vi "New Folder.vi"(8 "error in (no error)":errorcluster, 11 "folder name":string) -> (0 "error out":errorcluster, 3 "Folder Item out":refnum<class "Folder Item.lvclass">)   [LabVIEW 2020, in "BetterDragAndDropDemo.lvlib" / "Folder Item.lvclass"]
uses:
  Folder Item.lvclass
  Folder Item.lvclass/Folder Item.ctl
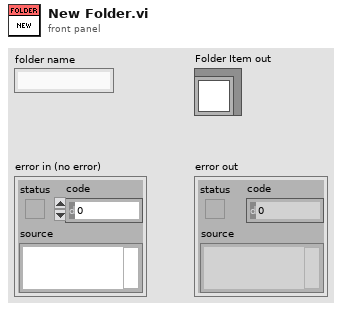
[diagram p1: front panel]
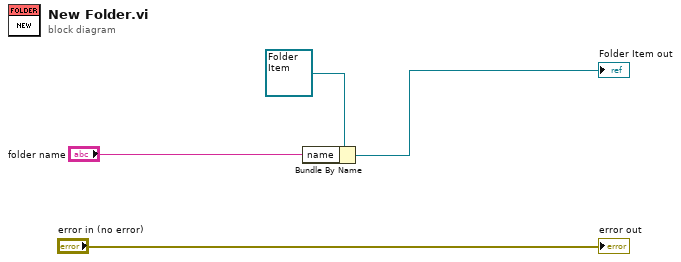
[diagram p0: block diagram]
diagram:
  n1 = Bundle By Name(cluster=refnum<class "Folder Item.lvclass"> refnum ("Folder Item out"), "name"="folder name") -> (→"Folder Item out":refnum<class "Folder Item.lvclass">)
  "error out" <- "error in (no error)"
